vi "Store Built Message.vi"(4 "Message Paths":T1, 8 "error in (no error)":errorcluster, 11 "LV-Protoc in":refnum<class "LV-Protoc.lvclass">) -> (0 "error out":errorcluster, 3 "LV-Protoc out":refnum<class "LV-Protoc.lvclass">)   [LabVIEW 2020, in "LV-Protoc.lvlib" / "LV-Protoc.lvclass"]
uses:
  LV-Protoc.lvclass
  Message Paths.ctl
  LV-Protoc.lvclass/LV-Protoc.ctl
  LV-Protoc.lvlib
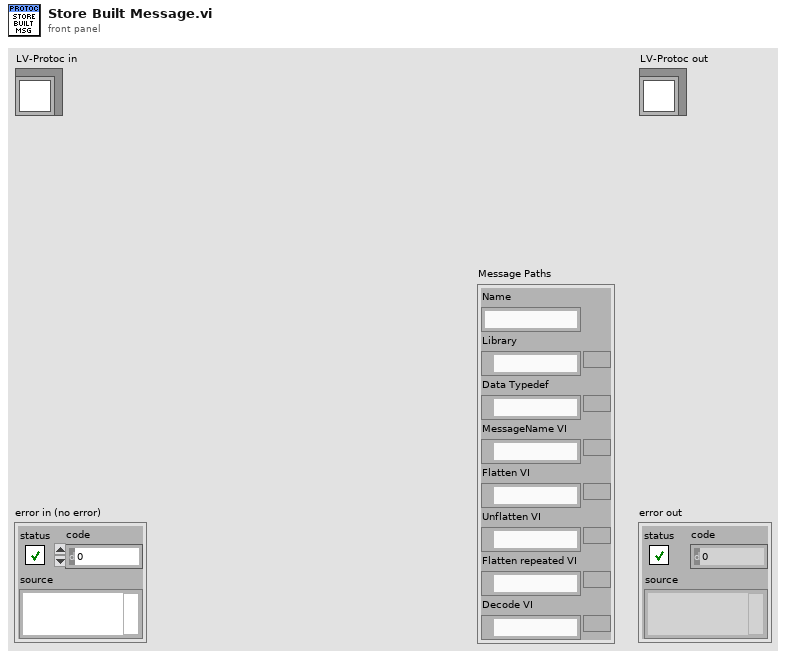
[diagram p1: front panel]
types:
  T1 = typedef "LV-Protoc.lvlib/Message Paths.ctl" = cluster{"Name":string, "Library":path, "Data Typedef":path, "MessageName VI":path, "Flatten VI":path, "Unflatten VI":path, "Flatten repeated VI":path, "Decode VI":path}
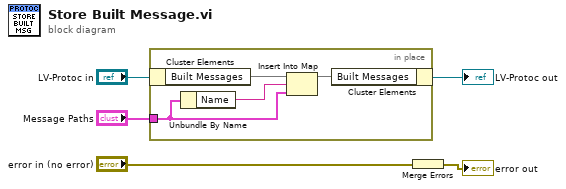
[diagram p0: block diagram]
diagram:
  n1 = in-place {
    in-place-border: "Message Paths" -> [w7]
    n2 = in-place-cluster #1("LV-Protoc in") -> ("Built Messages"=w9:map{string, T1})
    n3 = Unbundle By Name(w7) -> ("Name"=w8:string)
    n4 = Insert Into Map(map in=w9, key=w8, value=w7) -> (map out=w6:map{string, T1})  [unwired: 2 out]
    n5 = in-place-cluster #1("Built Messages"=w6) -> (→"LV-Protoc out":refnum<class "LV-Protoc.lvclass">)
  }
  n6 = Merge Errors("error in (no error)") -> (→"error out":errorcluster)
